vi "Stage_move_axis.vi"(7 "Direction true means positive increment":bool, 8 "error in (no error)":errorcluster, 9 "Distance micrometer":dbl, 10 "Axes Select":u16(ring) items=["X", "Y", "Z"], 11 "reference IN":refnum<k7>) -> (0 "error OUT":errorcluster, 3 "reference OUT":refnum<k7>)   [LabVIEW 2020]
uses:
  typedefs/typedef_boundaries.ctl
  Global stage boundaries.vi
panel:
  out "Stage boundary positions":T1={"X lower bound"=-40.0, "X upper bound"=2.6, "Y lower bound"=4.66, "Y upper bound "=12.78, "Z lower bound"=-0.001, "Z upper bound "=8.0}
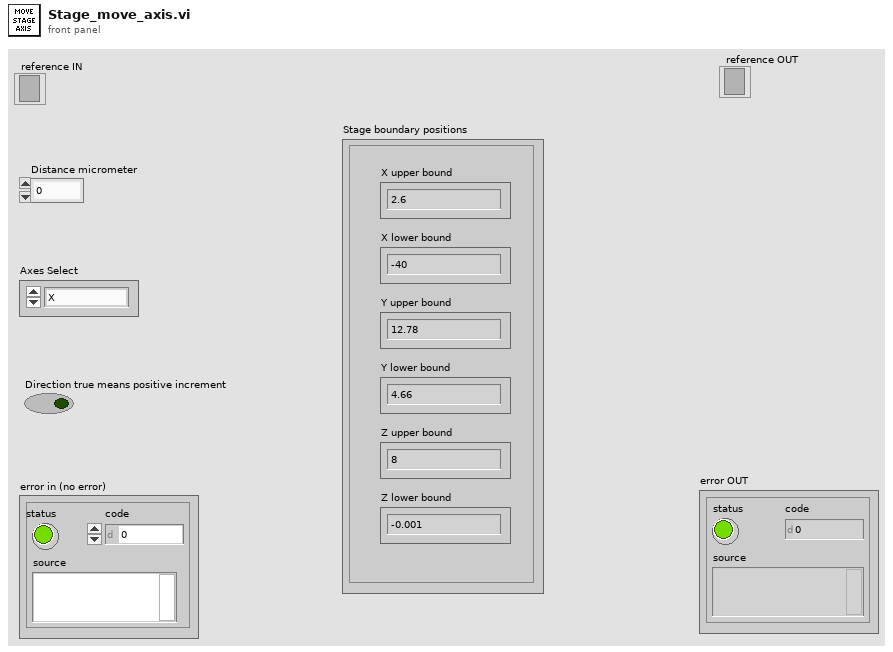
[diagram p1: front panel]
types:
  T1 = typedef "typedef_boundaries.ctl" = cluster{"X lower bound":dbl, "X upper bound":dbl, "Y lower bound":dbl, "Y upper bound ":dbl, "Z lower bound":dbl, "Z upper bound ":dbl}
  T2 = typedef "typedef_stage_position.ctl" = cluster{"X Position":dbl, "Y Position":dbl, "Z Position":dbl}
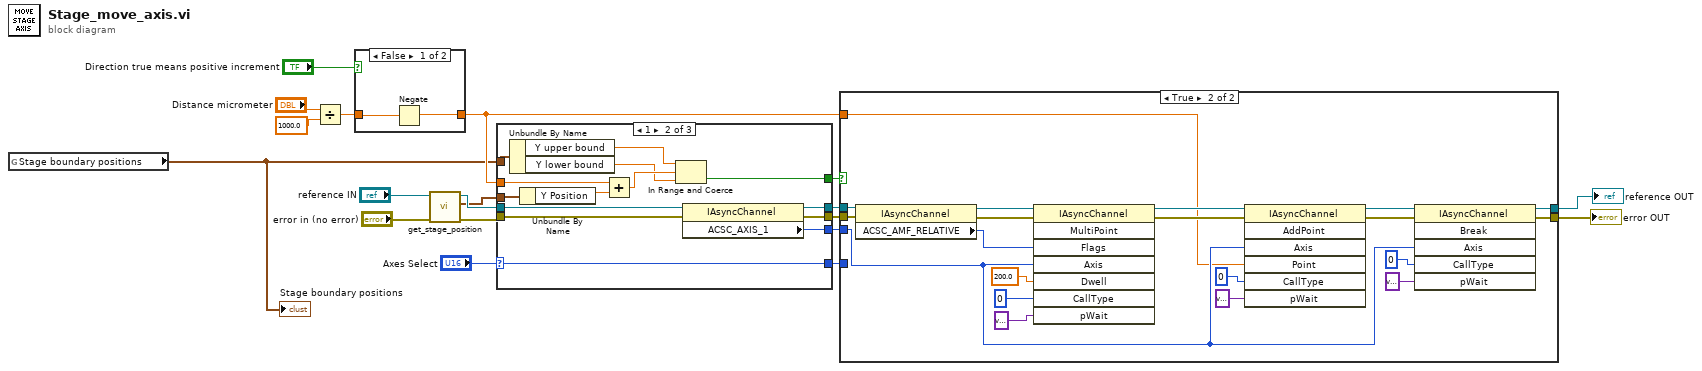
[diagram p0: block diagram]
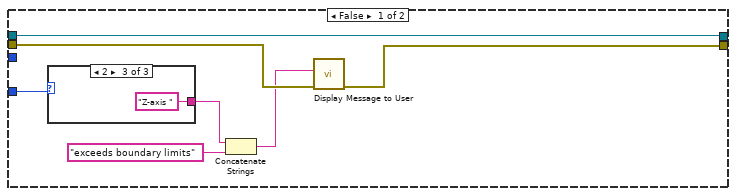
[diagram p2: hidden frame]
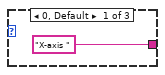
[diagram p3: hidden frame]
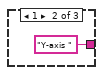
[diagram p4: hidden frame]
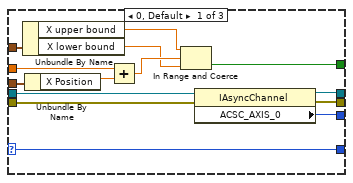
[diagram p6: hidden frame]
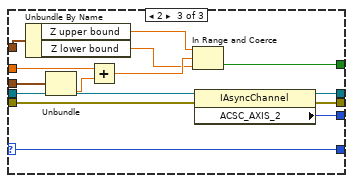
[diagram p7: hidden frame]
diagram:
  n1 = global read "Global stage boundaries.vi" "Stage boundary positions"() -> (w1:T1)
  "Stage boundary positions" <- w1
  n2 = Divide(x="Distance micrometer", y=1000.0) -> (x/y=w10:dbl)
  n3 = case shown="False" "Direction true means positive increment" {
    tunnel: w10 -> [w20 w22]
    tunnel: [w21 w22] -> w5
    frame False {
      n4 = Negate(x=w20) -> (-x=w21:dbl)
    }
    frame True {
    }
  }
  n5 = call "get_stage_position.vi"("error IN"="error in (no error)", "reference IN"="reference IN") -> ("error OUT"=w6:errorcluster, "Stage position OUT"=w2:T2, "reference OUT"=w7:refnum<k7>)  [unwired: 7 in]
  n6 = case shown="1" "Axes Select" {
    selector: "Axes Select" -> [w26 w40 w56]
    tunnel: [w34 w50 w64] -> w19
    tunnel: [w33 w49 w63] -> w18
    tunnel: [w32 w48 w62] -> w17
    tunnel: w7 -> [w36 w47 w61]
    tunnel: w6 -> [w35 w46 w60]
    tunnel: w2 -> [w31 w43 w55]
    tunnel: w5 -> [w30 w42 w58]
    tunnel: [w27 w41 w57] -> w4
    tunnel: [w26 w40 w56] -> w3
    tunnel: w1 -> [w25 w39 w53]
    frame 0, Default {
      n7 = Unbundle By Name(w25) -> ("X upper bound"=w24:dbl, "X lower bound"=w23:dbl)
      n8 = Unbundle By Name(w31) -> ("X Position"=w29:dbl)
      n9 = Add(x=w30, y=w29) -> (x+y=w28:dbl)
      n10 = In Range and Coerce(upper limit=w24, x=w28, lower limit=w23) -> (In Range?=w27:bool)  [unwired: 1 out]
      n11 = property class="IAsyncChannel"(reference=w36, error in=w35) -> (reference out=w34:refnum<k7>, error out=w33:errorcluster, "ACSC_AXIS_0"=w32:i32)
    }
    frame 1 {
      n12 = Unbundle By Name(w39) -> ("Y upper bound"=w38:dbl, "Y lower bound"=w37:dbl)
      n13 = Unbundle By Name(w43) -> ("Y Position"=w45:dbl)
      n14 = Add(x=w42, y=w45) -> (x+y=w44:dbl)
      n15 = In Range and Coerce(upper limit=w38, x=w44, lower limit=w37) -> (In Range?=w41:bool)  [unwired: 1 out]
      n16 = property class="IAsyncChannel"(reference=w47, error in=w46) -> (reference out=w50:refnum<k7>, error out=w49:errorcluster, "ACSC_AXIS_1"=w48:i32)
    }
    frame 2 {
      n17 = Unbundle By Name(w53) -> ("Z upper bound"=w52:dbl, "Z lower bound"=w51:dbl)
      n18 = Unbundle(w55) -> ("Z Position"=w54:dbl)  [unwired: 2 out]
      n19 = Add(x=w58, y=w54) -> (x+y=w59:dbl)
      n20 = In Range and Coerce(upper limit=w52, x=w59, lower limit=w51) -> (In Range?=w57:bool)  [unwired: 1 out]
      n21 = property class="IAsyncChannel"(reference=w61, error in=w60) -> (reference out=w64:refnum<k7>, error out=w63:errorcluster, "ACSC_AXIS_2"=w62:i32)
    }
  }
  n22 = case shown="True" w4 {
    tunnel: w19 -> [w71 w82]
    tunnel: w18 -> [w70 w81]
    tunnel: w17 -> [_ w80]
    tunnel: [w71 w77] -> w16
    tunnel: [w69 w76] -> w14
    tunnel: w5 -> [_ w75]
    tunnel: w3 -> [w66 _]
    frame False {
      n23 = case shown="2" w66 {
        tunnel: ["X-axis " "Y-axis " "Z-axis "] -> w65
        frame 0, Default {
        }
        frame 1 {
        }
        frame 2 {
        }
      }
      n24 = Concatenate Strings(w65, "exceeds boundary limits") -> (w67:string)
      n25 = call "Display Message to User"("error in (no error)"=w70, "Message"=w67) -> ("error out"=w69:errorcluster)  [unwired: 8 in, 1 out]
    }
    frame True {
      n26 = property class="IAsyncChannel"(reference=w82, error in=w81) -> (reference out=w94:refnum<k7>, error out=w93:errorcluster, "ACSC_AMF_RELATIVE"=w90:i32)
      n27 = invoke class="IAsyncChannel" method="MultiPoint"(reference=w94, error in=w93, "Flags"=w90, "Axis"=w80, "Dwell"=200.0, "CallType"=u64 0, "pWait"=variant) -> (reference out=w89:refnum<k7>, error out=w88:errorcluster)  [unwired: 1 in, 6 out]
      n28 = invoke class="IAsyncChannel" method="AddPoint"(reference=w89, error in=w88, "Axis"=w80, "Point"=w75, "CallType"=u64 0, "pWait"=variant) -> (reference out=w84:refnum<k7>, error out=w83:errorcluster)  [unwired: 1 in, 5 out]
      n29 = invoke class="IAsyncChannel" method="Break"(reference=w84, error in=w83, "Axis"=w80, "CallType"=u64 0, "pWait"=variant) -> (reference out=w77:refnum<k7>, error out=w76:errorcluster)  [unwired: 1 in, 4 out]
    }
  }
  "reference OUT" <- w16
  "error OUT" <- w14
